vi "WPI_MXP_Grab Mutex.vi"(2 "error in":errorcluster) -> (0 "error out":errorcluster, 1 "semaphore out":T1)   [LabVIEW 2017]
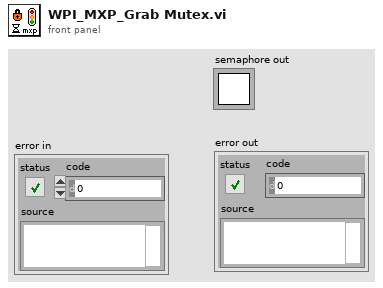
[diagram p1: front panel]
types:
  T1 = typedef "Semaphore RefNum" = refnum<k1>
  T2 = enum16{"Add", "Remove", "Acquire All", "Release All"}
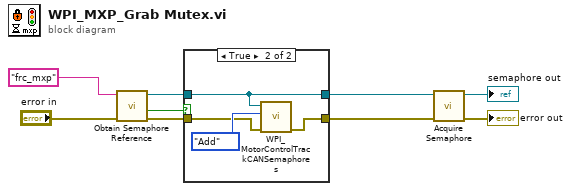
[diagram p0: block diagram]
diagram:
  n1 = call <vilib>:"Obtain Semaphore Reference.vi"("error in (no error)"="error in", "name (unnamed)"="frc_mxp") -> ("error out"=w4:errorcluster, "created new"=w5:bool, "semaphore"=w3:T1)  [unwired: 3 in]
  n2 = case shown="True" w5 {
    tunnel: w4 -> [w10 w13]
    tunnel: w3 -> [w11 w14]
    tunnel: [w11 w14] -> w2
    tunnel: [w10 w12] -> w1
    frame False {
    }
    frame True {
      n3 = call <vilib>:"WPI_MotorControlTrackCANSemaphores.vi"("error in (no error)"=w13, "Operation"=T2."Add", "semaphore"=w14) -> ("error out"=w12:errorcluster)  [unwired: 8 in]
    }
  }
  n4 = call <vilib>:"Acquire Semaphore.vi"("error in (no error)"=w1, "semaphore"=w2) -> ("error out"=→"error out":errorcluster, "semaphore out"=→"semaphore out":T1)  [unwired: 3 in, 1 out]
